vi "3D Numeric Integration.vi"(2 "integration method":T1 items=["Trapezoidal Rule", "Simpson's Rule", "Simpson's 3/8 Rule", "Bode Rule"], 3 "interval size":cluster{"dx":dbl, "dy":dbl, "dz":dbl}={"dx"=1.0, "dy"=1.0, "dz"=1.0}, 4 "Input Array":dbl[][][](array[numeric])) -> (0 "error":i32, 1 "result":dbl)   [LabVIEW 2017, in "NI_AALPro.lvlib"]
doc: "Performs numeric integration on the <B>Input Array</B> using one of four popular numeric integration methods. \n\nWire data to the <B>Input Array</B> input to determine the polymorphic instance to use or manually select the instance."
uses:
  NI_AALPro.lvlib
  Integral Method.ctl
  <resource>/lvanlys.dll
panel:
  # "3D Numeric Integration"
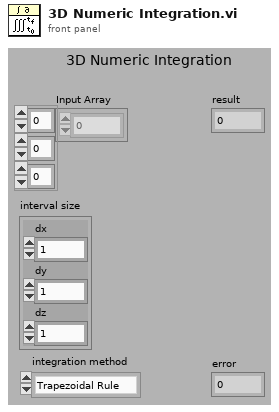
[diagram p1: front panel]
types:
  T1 = typedef "NI_AALPro.lvlib/Integral Method.ctl" = i32
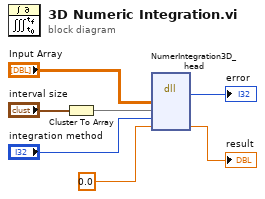
[diagram p0: block diagram]
diagram:
  n1 = Cluster To Array(cluster="interval size") -> (array=w2:dbl[])
  n2 = dll-call lib="C:/Program Files (x86)/National Instruments/LabVIEW 2017/resource/lvanlys.*" fn="NumerIntegration3D_head"("xHandle"="Input Array", "dx"=w2, "choice"="integration method", "result"=0.0) -> (→"error":i32, "result"=→"result":dbl)  [unwired: 4 in, 4 out]
